vi "ELVIS III v1.0 Enable Encoder.vi"(8 "error in (no error)":errorcluster, 9 "Enable":bool, 10 "Channel":T1, 11 "myRIO Ref In":T2) -> (0 "error out":errorcluster, 3 "myRIO Ref Out":T2)   [LabVIEW 2021]
uses:
  <vilib>/myRIO/Common/Instrument Driver Framework/Utilities/typedefs/myRIO v1.0 Reference.ctl
  <vilib>/myRIO/Common/Instrument Driver Framework/Utilities/typedefs/Generic FPGA Reference.ctl
  <vilib>/myRIO/Common/Instrument Driver Framework/myRIO v1.0/Encoder/typedefs/Encoder Channels Enum.ctl
  <vilib>/myRIO/Common/Instrument Driver Framework/ELVIS III v1.0/Encoder/typedefs/ELVIS III Encoder Channels FPGA Reference.ctl
  <vilib>/rvi/errors/niLvFpgaAdjustHostInterfaceError.vi
  <vilib>/rvi/interface/nirviReadWriteControl/nirviReadWriteControl.xnode
  <vilib>/rvi/interface/Simulation/niFpgaSimulationCallBeginRW.vi
  NiFpgaLv.dll
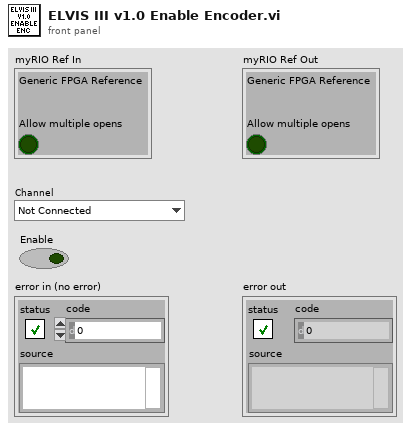
[diagram p1: front panel]
types:
  T1 = typedef "Encoder Channels Enum.ctl" = enum16{"Not Connected", "C/ENC0", "C/ENC1", "A/ENC", "A/ENC0", "A/ENC1", "A/ENC2", "A/ENC3", "A/ENC4", "A/ENC5", "A/ENC6", "A/ENC7", "A/ENC8", "A/ENC9", "B/ENC", "B/ENC0", "B/ENC1", "B/ENC2", "B/ENC3", "B/ENC4", "B/ENC5", "B/ENC6", "B/ENC7", "B/ENC8", "B/ENC9", "DIO/ENC0", "DIO/ENC1", "DIO/ENC2", "DIO/ENC3", "DIO/ENC4"}
  T2 = typedef "myRIO v1.0 Reference.ctl" = cluster{"Generic FPGA Reference":T3, "Allow multiple opens":bool}
  T3 = typedef "Generic FPGA Reference.ctl" = refnum<k20>
  T4 = typedef "ELVIS III Encoder Channels FPGA Reference.ctl" = refnum<k20>
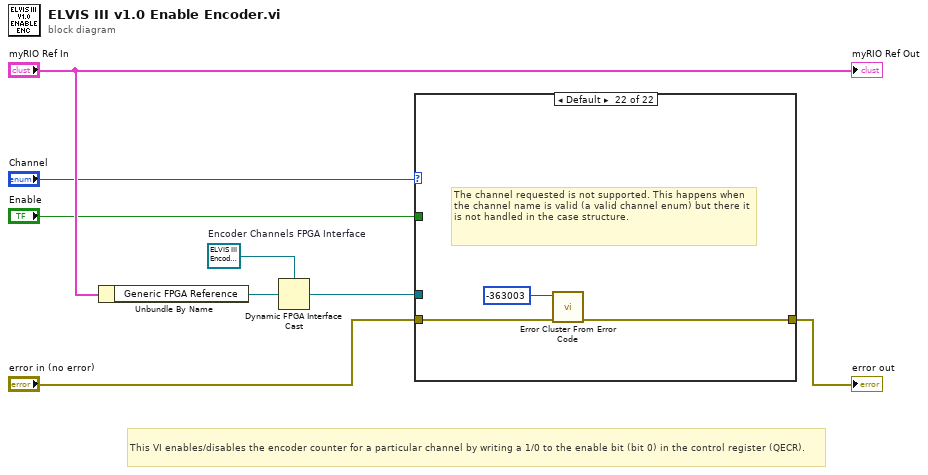
[diagram p0: block diagram]
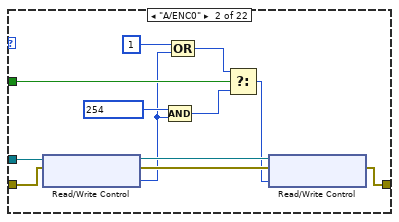
[diagram p3: hidden frame]
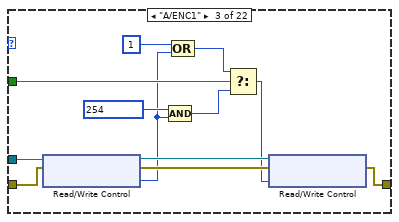
[diagram p4: hidden frame]
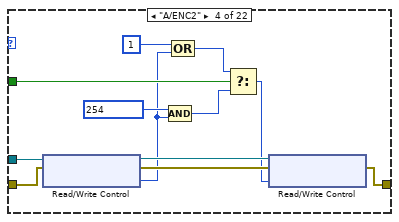
[diagram p5: hidden frame]
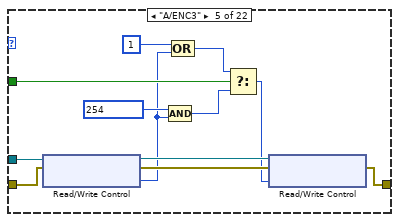
[diagram p6: hidden frame]
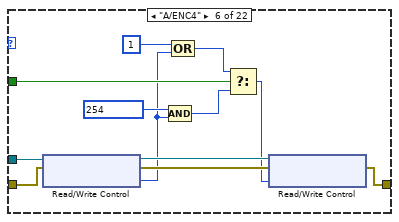
[diagram p7: hidden frame]
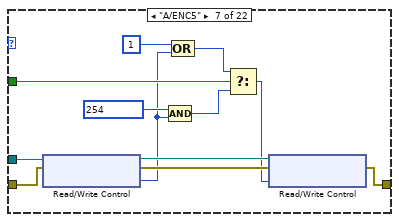
[diagram p8: hidden frame]
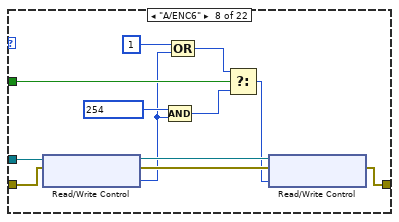
[diagram p9: hidden frame]
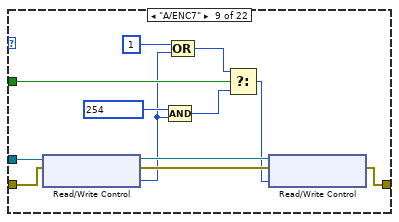
[diagram p10: hidden frame]
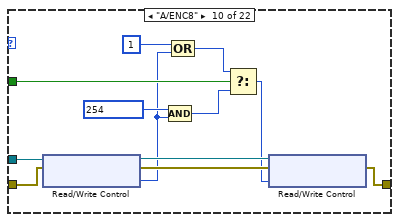
[diagram p11: hidden frame]
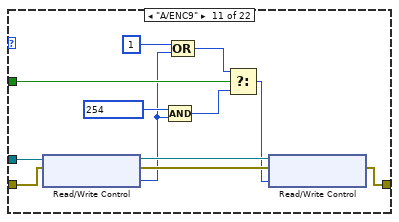
[diagram p12: hidden frame]
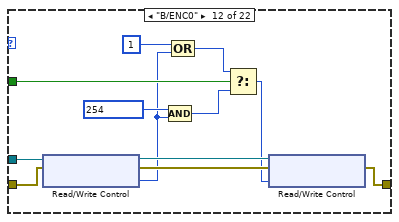
[diagram p13: hidden frame]
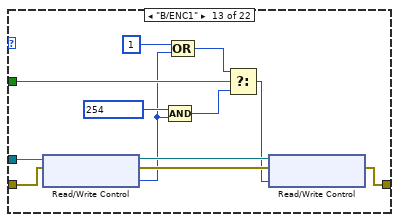
[diagram p14: hidden frame]
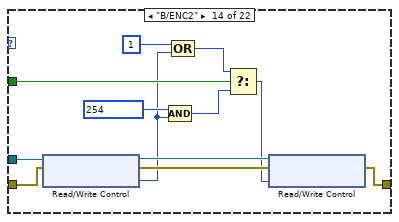
[diagram p15: hidden frame]
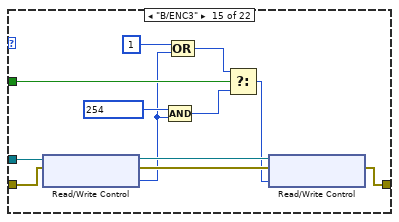
[diagram p16: hidden frame]
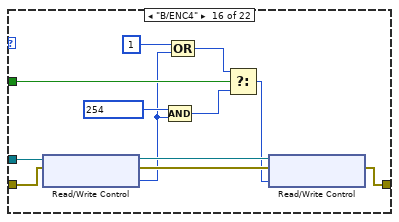
[diagram p17: hidden frame]
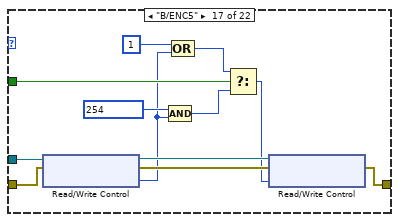
[diagram p18: hidden frame]
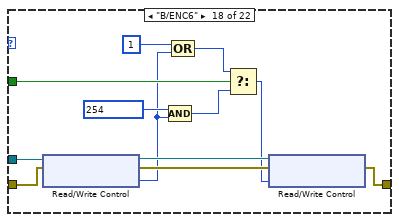
[diagram p19: hidden frame]
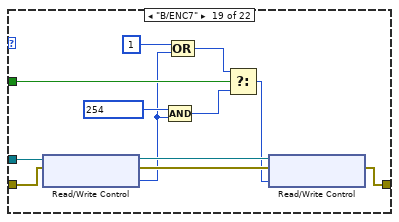
[diagram p20: hidden frame]
diagram:
  w8 = T4 refnum  # Encoder Channels FPGA Interface
  # "This VI enables/disables the encoder counter for a particular channel by writing a 1/0 to the enable bit (bit 0) in the control register (QECR)."
  n1 = Unbundle By Name("myRIO Ref In") -> ("Generic FPGA Reference"=w7:T3)
  n2 = Dynamic FPGA Interface Cast(Session In=w8, Type=w7) -> (Session Out=w5:T4)
  n3 = case shown="Default" "Channel" {
    tunnel: "error in (no error)" -> [w9 w15 w27 w39 w51 w63 w75 w87 w99 w111 w123 w135 w147 w159 w171 w183 w195 w207 w219 w231 w243 w250]
    tunnel: [w9 w13 w25 w37 w49 w61 w73 w85 w97 w109 w121 w133 w145 w157 w169 w181 w193 w205 w217 w229 w241 w251] -> w1
    tunnel: w5 -> [_ w16 w28 w40 w52 w64 w76 w88 w100 w112 w124 w136 w148 w160 w172 w184 w196 w208 w220 w232 w244 _]
    tunnel: "Enable" -> [_ w17 w29 w41 w53 w65 w77 w89 w101 w113 w125 w137 w149 w161 w173 w185 w197 w209 w221 w233 w245 _]
    frame "Not Connected" {
    }
    frame "A/ENC0" {
      n4 = xnode "Read/Write Control"("FPGA VI Reference In"=w16, "error in"=w15) -> ("FPGA VI Reference Out"=w12:T4, "error out"=w14:errorcluster, "ENC.A_0.CNFG"=w10:u8)
      n5 = Compound Arithmetic op=AND(u8 254, w10) -> (w21:u8)
      n6 = Compound Arithmetic op=OR(u8 1, w10) -> (w19:u8)
      n7 = Select(t=w19, s=w17, f=w21) -> (s? t:f=w11:u8)
      n8 = xnode "Read/Write Control"("FPGA VI Reference In"=w12, "error in"=w14, "ENC.A_0.CNFG"=w11) -> ("error out"=w13:errorcluster)  [unwired: 1 out]
    }
    frame "A/ENC1" {
      n9 = xnode "Read/Write Control"("FPGA VI Reference In"=w28, "error in"=w27) -> ("FPGA VI Reference Out"=w24:T4, "error out"=w26:errorcluster, "ENC.A_1.CNFG"=w22:u8)
      n10 = Compound Arithmetic op=AND(u8 254, w22) -> (w33:u8)
      n11 = Compound Arithmetic op=OR(u8 1, w22) -> (w31:u8)
      n12 = Select(t=w31, s=w29, f=w33) -> (s? t:f=w23:u8)
      n13 = xnode "Read/Write Control"("FPGA VI Reference In"=w24, "error in"=w26, "ENC.A_1.CNFG"=w23) -> ("error out"=w25:errorcluster)  [unwired: 1 out]
    }
    frame "A/ENC2" {
      n14 = xnode "Read/Write Control"("FPGA VI Reference In"=w40, "error in"=w39) -> ("FPGA VI Reference Out"=w36:T4, "error out"=w38:errorcluster, "ENC.A_2.CNFG"=w34:u8)
      n15 = Compound Arithmetic op=AND(u8 254, w34) -> (w45:u8)
      n16 = Compound Arithmetic op=OR(u8 1, w34) -> (w43:u8)
      n17 = Select(t=w43, s=w41, f=w45) -> (s? t:f=w35:u8)
      n18 = xnode "Read/Write Control"("FPGA VI Reference In"=w36, "error in"=w38, "ENC.A_2.CNFG"=w35) -> ("error out"=w37:errorcluster)  [unwired: 1 out]
    }
    frame "A/ENC3" {
      n19 = xnode "Read/Write Control"("FPGA VI Reference In"=w52, "error in"=w51) -> ("FPGA VI Reference Out"=w48:T4, "error out"=w50:errorcluster, "ENC.A_3.CNFG"=w46:u8)
      n20 = Compound Arithmetic op=AND(u8 254, w46) -> (w57:u8)
      n21 = Compound Arithmetic op=OR(u8 1, w46) -> (w55:u8)
      n22 = Select(t=w55, s=w53, f=w57) -> (s? t:f=w47:u8)
      n23 = xnode "Read/Write Control"("FPGA VI Reference In"=w48, "error in"=w50, "ENC.A_3.CNFG"=w47) -> ("error out"=w49:errorcluster)  [unwired: 1 out]
    }
    frame "A/ENC4" {
      n24 = xnode "Read/Write Control"("FPGA VI Reference In"=w64, "error in"=w63) -> ("FPGA VI Reference Out"=w60:T4, "error out"=w62:errorcluster, "ENC.A_4.CNFG"=w58:u8)
      n25 = Compound Arithmetic op=AND(u8 254, w58) -> (w69:u8)
      n26 = Compound Arithmetic op=OR(u8 1, w58) -> (w67:u8)
      n27 = Select(t=w67, s=w65, f=w69) -> (s? t:f=w59:u8)
      n28 = xnode "Read/Write Control"("FPGA VI Reference In"=w60, "error in"=w62, "ENC.A_4.CNFG"=w59) -> ("error out"=w61:errorcluster)  [unwired: 1 out]
    }
    frame "A/ENC5" {
      n29 = xnode "Read/Write Control"("FPGA VI Reference In"=w76, "error in"=w75) -> ("FPGA VI Reference Out"=w72:T4, "error out"=w74:errorcluster, "ENC.A_5.CNFG"=w70:u8)
      n30 = Compound Arithmetic op=AND(u8 254, w70) -> (w81:u8)
      n31 = Compound Arithmetic op=OR(u8 1, w70) -> (w79:u8)
      n32 = Select(t=w79, s=w77, f=w81) -> (s? t:f=w71:u8)
      n33 = xnode "Read/Write Control"("FPGA VI Reference In"=w72, "error in"=w74, "ENC.A_5.CNFG"=w71) -> ("error out"=w73:errorcluster)  [unwired: 1 out]
    }
    frame "A/ENC6" {
      n34 = xnode "Read/Write Control"("FPGA VI Reference In"=w88, "error in"=w87) -> ("FPGA VI Reference Out"=w84:T4, "error out"=w86:errorcluster, "ENC.A_6.CNFG"=w82:u8)
      n35 = Compound Arithmetic op=AND(u8 254, w82) -> (w93:u8)
      n36 = Compound Arithmetic op=OR(u8 1, w82) -> (w91:u8)
      n37 = Select(t=w91, s=w89, f=w93) -> (s? t:f=w83:u8)
      n38 = xnode "Read/Write Control"("FPGA VI Reference In"=w84, "error in"=w86, "ENC.A_6.CNFG"=w83) -> ("error out"=w85:errorcluster)  [unwired: 1 out]
    }
    frame "A/ENC7" {
      n39 = xnode "Read/Write Control"("FPGA VI Reference In"=w100, "error in"=w99) -> ("FPGA VI Reference Out"=w96:T4, "error out"=w98:errorcluster, "ENC.A_7.CNFG"=w94:u8)
      n40 = Compound Arithmetic op=AND(u8 254, w94) -> (w105:u8)
      n41 = Compound Arithmetic op=OR(u8 1, w94) -> (w103:u8)
      n42 = Select(t=w103, s=w101, f=w105) -> (s? t:f=w95:u8)
      n43 = xnode "Read/Write Control"("FPGA VI Reference In"=w96, "error in"=w98, "ENC.A_7.CNFG"=w95) -> ("error out"=w97:errorcluster)  [unwired: 1 out]
    }
    frame "A/ENC8" {
      n44 = xnode "Read/Write Control"("FPGA VI Reference In"=w112, "error in"=w111) -> ("FPGA VI Reference Out"=w108:T4, "error out"=w110:errorcluster, "ENC.A_8.CNFG"=w106:u8)
      n45 = Compound Arithmetic op=AND(u8 254, w106) -> (w117:u8)
      n46 = Compound Arithmetic op=OR(u8 1, w106) -> (w115:u8)
      n47 = Select(t=w115, s=w113, f=w117) -> (s? t:f=w107:u8)
      n48 = xnode "Read/Write Control"("FPGA VI Reference In"=w108, "error in"=w110, "ENC.A_8.CNFG"=w107) -> ("error out"=w109:errorcluster)  [unwired: 1 out]
    }
    frame "A/ENC9" {
      n49 = xnode "Read/Write Control"("FPGA VI Reference In"=w124, "error in"=w123) -> ("FPGA VI Reference Out"=w120:T4, "error out"=w122:errorcluster, "ENC.A_9.CNFG"=w118:u8)
      n50 = Compound Arithmetic op=AND(u8 254, w118) -> (w129:u8)
      n51 = Compound Arithmetic op=OR(u8 1, w118) -> (w127:u8)
      n52 = Select(t=w127, s=w125, f=w129) -> (s? t:f=w119:u8)
      n53 = xnode "Read/Write Control"("FPGA VI Reference In"=w120, "error in"=w122, "ENC.A_9.CNFG"=w119) -> ("error out"=w121:errorcluster)  [unwired: 1 out]
    }
    frame "B/ENC0" {
      n54 = xnode "Read/Write Control"("FPGA VI Reference In"=w136, "error in"=w135) -> ("FPGA VI Reference Out"=w132:T4, "error out"=w134:errorcluster, "ENC.B_0.CNFG"=w130:u8)
      n55 = Compound Arithmetic op=AND(u8 254, w130) -> (w141:u8)
      n56 = Compound Arithmetic op=OR(u8 1, w130) -> (w139:u8)
      n57 = Select(t=w139, s=w137, f=w141) -> (s? t:f=w131:u8)
      n58 = xnode "Read/Write Control"("FPGA VI Reference In"=w132, "error in"=w134, "ENC.B_0.CNFG"=w131) -> ("error out"=w133:errorcluster)  [unwired: 1 out]
    }
    frame "B/ENC1" {
      n59 = xnode "Read/Write Control"("FPGA VI Reference In"=w148, "error in"=w147) -> ("FPGA VI Reference Out"=w144:T4, "error out"=w146:errorcluster, "ENC.B_1.CNFG"=w142:u8)
      n60 = Compound Arithmetic op=AND(u8 254, w142) -> (w153:u8)
      n61 = Compound Arithmetic op=OR(u8 1, w142) -> (w151:u8)
      n62 = Select(t=w151, s=w149, f=w153) -> (s? t:f=w143:u8)
      n63 = xnode "Read/Write Control"("FPGA VI Reference In"=w144, "error in"=w146, "ENC.B_1.CNFG"=w143) -> ("error out"=w145:errorcluster)  [unwired: 1 out]
    }
    frame "B/ENC2" {
      n64 = xnode "Read/Write Control"("FPGA VI Reference In"=w160, "error in"=w159) -> ("FPGA VI Reference Out"=w156:T4, "error out"=w158:errorcluster, "ENC.B_2.CNFG"=w154:u8)
      n65 = Compound Arithmetic op=AND(u8 254, w154) -> (w165:u8)
      n66 = Compound Arithmetic op=OR(u8 1, w154) -> (w163:u8)
      n67 = Select(t=w163, s=w161, f=w165) -> (s? t:f=w155:u8)
      n68 = xnode "Read/Write Control"("FPGA VI Reference In"=w156, "error in"=w158, "ENC.B_2.CNFG"=w155) -> ("error out"=w157:errorcluster)  [unwired: 1 out]
    }
    frame "B/ENC3" {
      n69 = xnode "Read/Write Control"("FPGA VI Reference In"=w172, "error in"=w171) -> ("FPGA VI Reference Out"=w168:T4, "error out"=w170:errorcluster, "ENC.B_3.CNFG"=w166:u8)
      n70 = Compound Arithmetic op=AND(u8 254, w166) -> (w177:u8)
      n71 = Compound Arithmetic op=OR(u8 1, w166) -> (w175:u8)
      n72 = Select(t=w175, s=w173, f=w177) -> (s? t:f=w167:u8)
      n73 = xnode "Read/Write Control"("FPGA VI Reference In"=w168, "error in"=w170, "ENC.B_3.CNFG"=w167) -> ("error out"=w169:errorcluster)  [unwired: 1 out]
    }
    frame "B/ENC4" {
      n74 = xnode "Read/Write Control"("FPGA VI Reference In"=w184, "error in"=w183) -> ("FPGA VI Reference Out"=w180:T4, "error out"=w182:errorcluster, "ENC.B_4.CNFG"=w178:u8)
      n75 = Compound Arithmetic op=AND(u8 254, w178) -> (w189:u8)
      n76 = Compound Arithmetic op=OR(u8 1, w178) -> (w187:u8)
      n77 = Select(t=w187, s=w185, f=w189) -> (s? t:f=w179:u8)
      n78 = xnode "Read/Write Control"("FPGA VI Reference In"=w180, "error in"=w182, "ENC.B_4.CNFG"=w179) -> ("error out"=w181:errorcluster)  [unwired: 1 out]
    }
    frame "B/ENC5" {
      n79 = xnode "Read/Write Control"("FPGA VI Reference In"=w196, "error in"=w195) -> ("FPGA VI Reference Out"=w192:T4, "error out"=w194:errorcluster, "ENC.B_5.CNFG"=w190:u8)
      n80 = Compound Arithmetic op=AND(u8 254, w190) -> (w201:u8)
      n81 = Compound Arithmetic op=OR(u8 1, w190) -> (w199:u8)
      n82 = Select(t=w199, s=w197, f=w201) -> (s? t:f=w191:u8)
      n83 = xnode "Read/Write Control"("FPGA VI Reference In"=w192, "error in"=w194, "ENC.B_5.CNFG"=w191) -> ("error out"=w193:errorcluster)  [unwired: 1 out]
    }
    frame "B/ENC6" {
      n84 = xnode "Read/Write Control"("FPGA VI Reference In"=w208, "error in"=w207) -> ("FPGA VI Reference Out"=w204:T4, "error out"=w206:errorcluster, "ENC.B_6.CNFG"=w202:u8)
      n85 = Compound Arithmetic op=AND(u8 254, w202) -> (w213:u8)
      n86 = Compound Arithmetic op=OR(u8 1, w202) -> (w211:u8)
      n87 = Select(t=w211, s=w209, f=w213) -> (s? t:f=w203:u8)
      n88 = xnode "Read/Write Control"("FPGA VI Reference In"=w204, "error in"=w206, "ENC.B_6.CNFG"=w203) -> ("error out"=w205:errorcluster)  [unwired: 1 out]
    }
    frame "B/ENC7" {
      n89 = xnode "Read/Write Control"("FPGA VI Reference In"=w220, "error in"=w219) -> ("FPGA VI Reference Out"=w216:T4, "error out"=w218:errorcluster, "ENC.B_7.CNFG"=w214:u8)
      n90 = Compound Arithmetic op=AND(u8 254, w214) -> (w225:u8)
      n91 = Compound Arithmetic op=OR(u8 1, w214) -> (w223:u8)
      n92 = Select(t=w223, s=w221, f=w225) -> (s? t:f=w215:u8)
      n93 = xnode "Read/Write Control"("FPGA VI Reference In"=w216, "error in"=w218, "ENC.B_7.CNFG"=w215) -> ("error out"=w217:errorcluster)  [unwired: 1 out]
    }
    frame "B/ENC8" {
      n94 = xnode "Read/Write Control"("FPGA VI Reference In"=w232, "error in"=w231) -> ("FPGA VI Reference Out"=w228:T4, "error out"=w230:errorcluster, "ENC.B_8.CNFG"=w226:u8)
      n95 = Compound Arithmetic op=AND(u8 254, w226) -> (w237:u8)
      n96 = Compound Arithmetic op=OR(u8 1, w226) -> (w235:u8)
      n97 = Select(t=w235, s=w233, f=w237) -> (s? t:f=w227:u8)
      n98 = xnode "Read/Write Control"("FPGA VI Reference In"=w228, "error in"=w230, "ENC.B_8.CNFG"=w227) -> ("error out"=w229:errorcluster)  [unwired: 1 out]
    }
    frame "B/ENC9" {
      n99 = xnode "Read/Write Control"("FPGA VI Reference In"=w244, "error in"=w243) -> ("FPGA VI Reference Out"=w240:T4, "error out"=w242:errorcluster, "ENC.B_9.CNFG"=w238:u8)
      n100 = Compound Arithmetic op=AND(u8 254, w238) -> (w249:u8)
      n101 = Compound Arithmetic op=OR(u8 1, w238) -> (w247:u8)
      n102 = Select(t=w247, s=w245, f=w249) -> (s? t:f=w239:u8)
      n103 = xnode "Read/Write Control"("FPGA VI Reference In"=w240, "error in"=w242, "ENC.B_9.CNFG"=w239) -> ("error out"=w241:errorcluster)  [unwired: 1 out]
    }
    frame Default {
      # "The channel requested is not supported. This happens when the channel name is valid (a valid channel enum) but there it is not handled in the case structure."
      n104 = call <vilib>:"Error Cluster From Error Code.vi"("error in (no error)"=w250, "error code (0)"=-363003) -> ("error out"=w251:errorcluster)  [unwired: 7 in]
    }
  }
  "error out" <- w1
  "myRIO Ref Out" <- "myRIO Ref In"
